vi "Initialize.vi"(7 "Serial Configuration":T1={"Baud Rate"=9600, "Parity"=0, "Data Bits"=8, "Stop Bits"=10, "Flow Control"=0} {"Flow Control" items=["None", "XON/XOFF", "RTS/CTS", "XON/XOFF & RTS/CTS", "DTR/DSR", "XON/XOFF & DTR/DSR"]; "Stop Bits" items=["1.0"=10, "1.5"=15, "2.0"=20]; "Data Bits" items=["7"=7, "8"=8]; "Parity" items=["None", "Odd", "Even", "Mark", "Space"]; "Baud Rate" items=["300"=300, "600"=600, "1200"=1200, "2400"=2400, "4800"=4800, "9600"=9600, "19200"=19200]}, 8 "error in (no error)":errorcluster, 9 "Reset (True)":bool=TRUE, 10 "ID Query (True)":bool=TRUE, 11 "VISA resource name":refnum<visa-resource-name>) -> (0 "error out":errorcluster, 3 "VISA resource name out":refnum<visa-resource-name>)   [LabVIEW 2015, in "IT6000C.lvlib"]
doc: "Establishes communication with the instrument and optionally performs an instrument identification query and/or an instrument reset. It also places the instrument in a default state needed for other instrument driver operations. Therefore, call this VI before calling other instrument driver VIs for this instrument. Generally, you need to call the <b>Initialize</b> VI only once at the beginning of an application."
uses:
  <instrlib>/IT6000C/IT6000C.lvlib
panel:
  # "(c) 2014 <Enter Company Name Here>.  ALL RIGHTS RESERVED."
  # "EDIT: Change control description to remove example text for buses not supported."
  # "EDIT: Serial settings must match those on the physical instrument.  Review user's manual to determine the correct Flow Control protocol for the instrument.  \"None\" is the least robust option for this setting, and could lead to unreliable data transmission."
  # "EDIT: If your instrument does not support ID query or Reset, remove the ID Query or Reset control from the front panel and delete the case structure with the ID Query or Reset code from the block diagram."
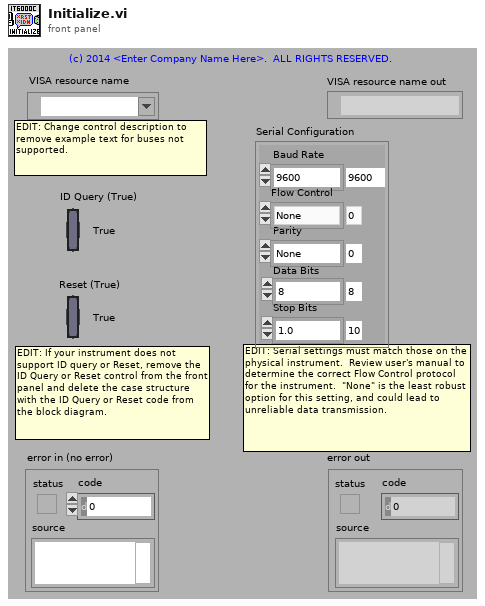
[diagram p1: front panel]
types:
  T1 = cluster{"Baud Rate":u32, "Parity":u16, "Data Bits":u16, "Stop Bits":u16, "Flow Control":u16}
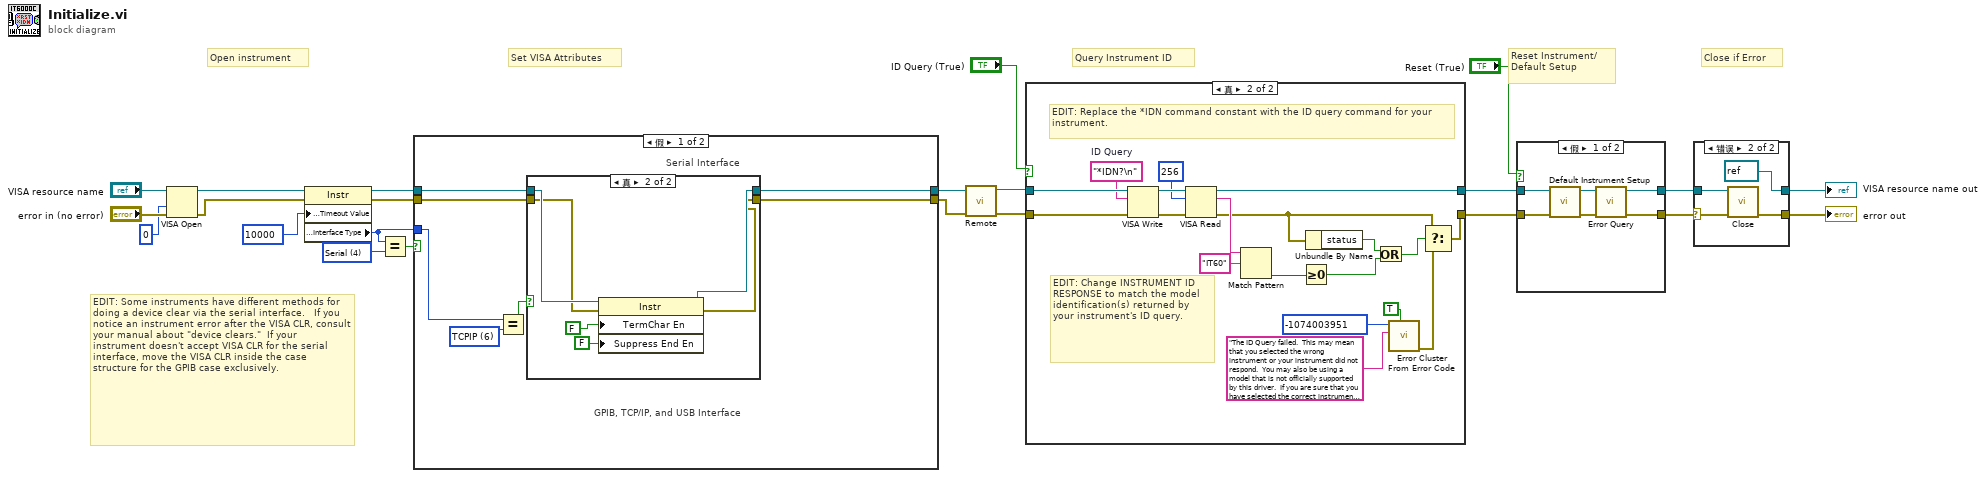
[diagram p0: block diagram]
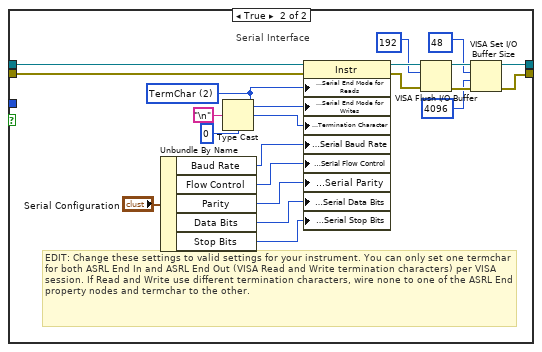
[diagram p3: hidden frame]
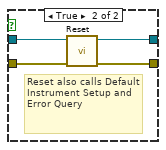
[diagram p5: hidden frame]
diagram:
  w13 = u16 4 items=["GPIB"=1, "VXI"=2, "GPIB-VXI"=3, "Serial"=4, "PXI"=5, "TCPIP"=6, "USB"=7] ("Interface Information:Interface Type")
  # "EDIT: Some instruments have different methods for doing a device clear via the serial interface.   If you notice an instrument error after the VISA CLR, consult your manual about \"device clears.\"  If your instrument doesn't accept VISA CLR for the serial interface, move the VISA CLR inside the case  structure for the GPIB case exclusively."
  # "Set VISA Attributes"
  # "Close if Error"
  # "Query Instrument ID"
  # "Reset Instrument/\nDefault Setup"
  # "Open instrument"
  n1 = VISA Open(access mode=u32 0, error in (no error)="error in (no error)", VISA resource name="VISA resource name") -> (VISA resource name=w11:refnum<visa-resource-name>, error out=w10:errorcluster)  [unwired: 2 in]
  n2 = property class="Instr"(reference=w11, error in=w10, "General Settings:Timeout Value"=u32 10000) -> (reference out=w16:refnum<visa-resource-name>, error out=w15:errorcluster, "Interface Information:Interface Type"=w1:u16)
  n3 = Equal?(x=w1, y=w13) -> (x = y?=w14:bool)
  n4 = case shown="假" w14 {
    tunnel: [w25 w56] -> w2
    tunnel: [w24 w53] -> w3
    tunnel: w16 -> [w27 w58]
    tunnel: w15 -> [w26 w59]
    tunnel: w1 -> [w28 _]
    frame False {
      w29 = u16 6 items=["GPIB"=1, "VXI"=2, "GPIB-VXI"=3, "Serial"=4, "PXI"=5, "TCPIP"=6, "USB"=7] ("Interface Information:Interface Type")
      # "Serial Interface"
      # "GPIB, TCP/IP, and USB Interface"
      n5 = Equal?(x=w28, y=w29) -> (x = y?=w30:bool)
      n6 = case shown="真" w30 {
        tunnel: w27 -> [w32 w35]
        tunnel: w26 -> [w31 w34]
        tunnel: [w32 w37] -> w25
        tunnel: [w31 w36] -> w24
        frame False {
        }
        frame True {
          n7 = property class="Instr"(reference=w35, error in=w34, "TermChar En"=FALSE, "Suppress End En"=FALSE ("Message Based Settings:Suppress End Enable")) -> (reference out=w37:refnum<visa-resource-name>, error out=w36:errorcluster)
        }
      }
    }
    frame True {
      w46 = u16 2 items=["None", "LastBit", "TermChar"] ("Serial Settings:Serial End Mode for Reads")
      # "EDIT: Change these settings to valid settings for your instrument. You can only set one termchar for both ASRL End In and ASRL End Out (VISA Read and Write termination characters) per VISA session. If Read and Write use different termination characters, wire none to one of the ASRL End property nodes and termchar to the other."
      # "Serial Interface"
      n8 = Unbundle By Name("Serial Configuration") -> ("Baud Rate"=w44:u32, "Flow Control"=w40:u16, "Parity"=w42:u16, "Data Bits"=w43:u16, "Stop Bits"=w39:u16)
      n9 = Type Cast(type=u8 0, x="\n" ("Line Feed Constant")) -> (*(type *) &x=w45:u8)
      n10 = property class="Instr"(reference=w58, error in=w59, "Serial Settings:Serial End Mode for Reads"=w46, "Serial Settings:Serial End Mode for Writes"=w46, "Message Based Settings:Termination Character"=w45, "Serial Settings:Serial Baud Rate"=w44, "Serial Settings:Serial Flow Control"=w40, "Serial Settings:Serial Parity"=w42, "Serial Settings:Serial Data Bits"=w43, "Serial Settings:Serial Stop Bits"=w39) -> (reference out=w52:refnum<visa-resource-name>, error out=w55:errorcluster)
      n11 = VISA Flush I/O Buffer(VISA resource name=w52, mask (16)=u16 192, error in (no error)=w55) -> (VISA resource name out=w57:refnum<visa-resource-name>, error out=w54:errorcluster)
      n12 = VISA Set I/O Buffer Size(VISA resource name=w57, mask (16)=u16 48, size (4096)=u32 4096 ("size (0)"), error in (no error)=w54) -> (VISA resource name out=w56:refnum<visa-resource-name>, error out=w53:errorcluster)
    }
  }
  n13 = call <instrlib>:"Remote.vi"("error in (no error)"=w3, "VISA resource name"=w2) -> ("error out"=w4:errorcluster, "VISA resource name out"=w5:refnum<visa-resource-name>)  [unwired: 8 in]
  n14 = case shown="真" "ID Query (True)" {
    tunnel: [w60 w80] -> w22
    tunnel: [w61 w77] -> w23
    tunnel: w5 -> [w61 w78]
    tunnel: w4 -> [w60 w79]
    frame False {
    }
    frame True {
      w71 = "*IDN?\n"  # ID Query
      # "EDIT: Replace the *IDN command constant with the ID query command for your instrument."
      # "EDIT: Change INSTRUMENT ID RESPONSE to match the model identification(s) returned by your instrument's ID query."
      n15 = VISA Write(VISA resource name=w78, write buffer=w71, error in (no error)=w79) -> (VISA resource name out=w75:refnum<visa-resource-name>, error out=w74:errorcluster)  [unwired: 1 out]
      n16 = VISA Read(VISA resource name=w75, byte count=u32 256, error in (no error)=w74) -> (VISA resource name out=w77:refnum<visa-resource-name>, read buffer=w76:string, error out=w65:errorcluster)  [unwired: 1 out]
      n17 = Match Pattern(string=w76, regular expression="IT60") -> (offset past match=w66:i32)  [unwired: 1 in, 3 out]
      n18 = Greater Or Equal To 0?(x=w66) -> (x >= 0?=w63:bool)
      n19 = Unbundle By Name(w65) -> ("status"=w64:bool)
      n20 = Or(x=w64, y=w63) -> (x .or. y?=w62:bool)
      n21 = call <vilib>:"Error Cluster From Error Code.vi"("show call chain? (False)"=TRUE, "error message (\"\")"="The ID Query failed.  This may mean that you selected the wrong instrument or your instrument did not respond.  You may also be using a model that is not officially supported by this driver.  If you are sure that you have selected the correct instrument and it is responding, try disabling the ID Query." ("Source (VI Name)"), "error code (0)"=-1074003951 ("Code")) -> ("error out"=w70:errorcluster)  [unwired: 6 in]
      n22 = Select(t=w65, s=w62, f=w70) -> (s? t:f=w80:errorcluster)
    }
  }
  n23 = case shown="假" "Reset (True)" {
    tunnel: w22 -> [w85 w87]
    tunnel: [w82 w90] -> w6
    tunnel: w23 -> [w86 w88]
    tunnel: [w83 w89] -> w7
    frame False {
      n24 = call <instrlib>:"Default Instrument Setup.vi"("error in (no error)"=w85, "VISA resource name"=w86) -> ("error out"=w81:errorcluster, "VISA resource name out"=w84:refnum<visa-resource-name>)  [unwired: 8 in]
      n25 = call <instrlib>:"Error Query.vi"("error in (no error)"=w81, "VISA resource name"=w84) -> ("error out"=w82:errorcluster, "VISA resource name out"=w83:refnum<visa-resource-name>)  [unwired: 6 in, 2 out]
    }
    frame True {
      # "Reset also calls Default Instrument Setup and Error Query"
      n26 = call <instrlib>:"Reset.vi"("error in (no error)"=w87, "VISA resource name"=w88) -> ("error out"=w90:errorcluster, "VISA resource name out"=w89:refnum<visa-resource-name>)  [unwired: 8 in]
    }
  }
  n27 = case shown="错误" w6 {
    selector: w6 -> [w91 w94]
    tunnel: w7 -> [w92 w95]
    tunnel: [w92 refnum<visa-resource-name> refnum ("VISA resource name out")] -> w9
    tunnel: [w91 w96] -> w8
    frame No Error {
    }
    frame Error {
      n28 = call <instrlib>:"Close.vi"("error in (no error)"=w94, "VISA resource name"=w95) -> ("error out"=w96:errorcluster)  [unwired: 9 in]
    }
  }
  "VISA resource name out" <- w9
  "error out" <- w8
